vi "DOConfigureCustomaPattern.vi"(0 "object in":refnum<class "AD2_DO_SDK.lvclass">, 2 "?":T1={"DO Trigger"={"secRun(0=Cont)"=0.0, "secWait"=0.0, "cRepeat(0=inf)"=0, "Repeat Trigger"=FALSE, "TrigrSrc"=enum."trigrsrcNone"}, "CustomData"=[{"Data"=[FALSE, TRUE, FALSE, FALSE, FALSE, FALSE, FALSE, FALSE, FALSE, FALSE, FALSE, FALSE, FALSE, FALSE, FALSE, FALSE, FALSE, FALSE, FALSE, FALSE, FALSE, FALSE], "Freq"=1000.0, "#Bits"=100, "Enable"=FALSE, "IdleState"=0}, {"Data"=[TRUE, TRUE, TRUE, TRUE, TRUE, FALSE, FALSE, FALSE, FALSE, FALSE, FALSE, FALSE, FALSE, FALSE, FALSE, FALSE, FALSE, FALSE, FALSE, FALSE, FALSE, FALSE], "Freq"=1000.0, "#Bits"=100, "Enable"=FALSE, "IdleState"=0}, {"Data"=[], "Freq"=0.0, "#Bits"=0, "Enable"=FALSE, "IdleState"=0}, {"Data"=[FALSE, FALSE, FALSE, FALSE, FALSE, FALSE, FALSE, FALSE, FALSE, FALSE, FALSE, FALSE, FALSE, FALSE, FALSE, FALSE, FALSE, FALSE, FALSE, FALSE, FALSE, FALSE, FALSE], "Freq"=0.0, "#Bits"=0, "Enable"=FALSE, "IdleState"=0}, {"Data"=[], "Freq"=0.0, "#Bits"=0, "Enable"=FALSE, "IdleState"=0}, {"Data"=[], "Freq"=0.0, "#Bits"=0, "Enable"=FALSE, "IdleState"=0}, {"Data"=[], "Freq"=0.0, "#Bits"=0, "Enable"=FALSE, "IdleState"=0}, {"Data"=[], "Freq"=0.0, "#Bits"=0, "Enable"=FALSE, "IdleState"=0}, {"Data"=[], "Freq"=0.0, "#Bits"=0, "Enable"=FALSE, "IdleState"=0}, {"Data"=[], "Freq"=0.0, "#Bits"=0, "Enable"=FALSE, "IdleState"=0}, {"Data"=[], "Freq"=0.0, "#Bits"=0, "Enable"=FALSE, "IdleState"=0}, {"Data"=[], "Freq"=0.0, "#Bits"=0, "Enable"=FALSE, "IdleState"=0}, {"Data"=[], "Freq"=0.0, "#Bits"=0, "Enable"=FALSE, "IdleState"=0}, {"Data"=[], "Freq"=0.0, "#Bits"=0, "Enable"=FALSE, "IdleState"=0}, {"Data"=[], "Freq"=0.0, "#Bits"=0, "Enable"=FALSE, "IdleState"=0}, {"Data"=[FALSE, FALSE, FALSE, FALSE, FALSE, FALSE, FALSE, FALSE, FALSE, FALSE, FALSE, FALSE, FALSE, FALSE, FALSE, FALSE, FALSE, FALSE, FALSE, FALSE, FALSE, FALSE, FALSE], "Freq"=0.0, "#Bits"=0, "Enable"=FALSE, "IdleState"=0}, {"Data"=[FALSE, FALSE, FALSE, FALSE, FALSE, FALSE, FALSE, FALSE, FALSE, FALSE, FALSE, FALSE, FALSE, FALSE, FALSE, FALSE, FALSE, FALSE, FALSE, FALSE, FALSE, FALSE, FALSE], "Freq"=0.0, "#Bits"=0, "Enable"=FALSE, "IdleState"=0}]}, 5 "error in (no error)":errorcluster) -> (14 "object out":refnum<class "AD2_DO_SDK.lvclass">, 19 "error out":errorcluster)   [LabVIEW 2023, in "AD2_DO_SDK.lvclass"]
uses:
  AD2_DO_SDK.lvclass
  DOConfigureCustomData.ctl
  DOTrigger.ctl
  AD2_WFG_SDK_class/AD2TriggerSources.ctl
  DOCustomData.ctl
  AD2_DO_SDK.lvclass/AD2_DO_SDK.ctl
  Olasdwf/Olasdwf.lvlib
  AD2_SDK_class/AD2_SDK.lvclass
panel:
  out "In Range?":bool
  out "pcountOfBitsMax out":u32
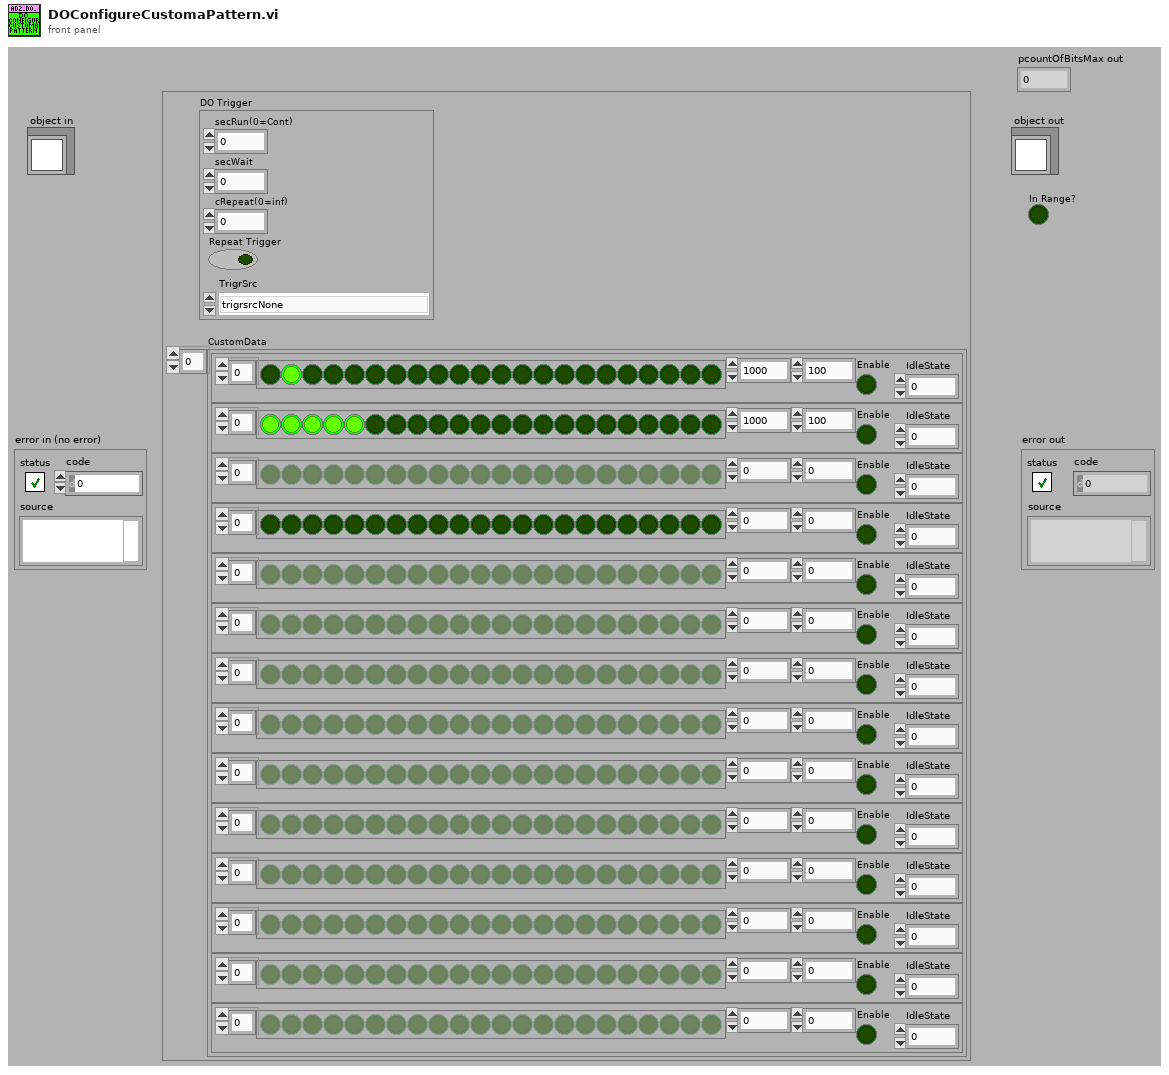
[diagram p1: front panel]
types:
  T1 = typedef "DOConfigureCustomData.ctl" = cluster{"DO Trigger":T2, "CustomData":T4}
  T2 = typedef "AD2_DO_SDK.lvclass/DOTrigger.ctl" = cluster{"secRun(0=Cont)":dbl, "secWait":dbl, "cRepeat(0=inf)":i32, "Repeat Trigger":bool, "TrigrSrc":T3}
  T3 = typedef "AD2_SDK.lvclass/AD2TriggerSources.ctl" = enum8{"trigrsrcNone", "trigsrcPC", "trigsrcDetectorAnalogIn", "trigsrcDetectorDigitalIn", "trigsrcAnalogIn", "trigsrcDigitalIn", "trigsrcDigitalOut", "trigsrcAnalogOut1", "trigsrcAnalogOut2", "trigsrcAnalogOut3", "trigsrcAnalogOut4", "trigsrcExternal1", "trigsrcExternal2", "trigsrcExternal3", "trigsrcExternal4", ""}
  T4 = typedef "AD2_DO_SDK.lvclass/DOCustomData.ctl" = cluster{"Data":bool[], "Freq":dbl, "#Bits":u32, "Enable":bool, "IdleState":u16}[]
  T5 = cluster{"NoHighBits":u32, "NoLowBits":u32, "NoInitialBits":u32, "Start High":bool}
  T6 = typedef "AD2_DO_SDK.lvclass/DOSingleCh.ctl" = cluster{"Ch Index":i32, "Enable":bool, "Clock DIvider":u32, "Type":i32, "DigitalOutOutput":u16, "IdleState":u16, "CounterData":cluster{"NoHighBits":u32, "NoLowBits":u32, "NoInitialBits":u32, "Start High":bool}, "Custom Data":cluster{"countOfBits":u32, "rgBits":u8[]}}
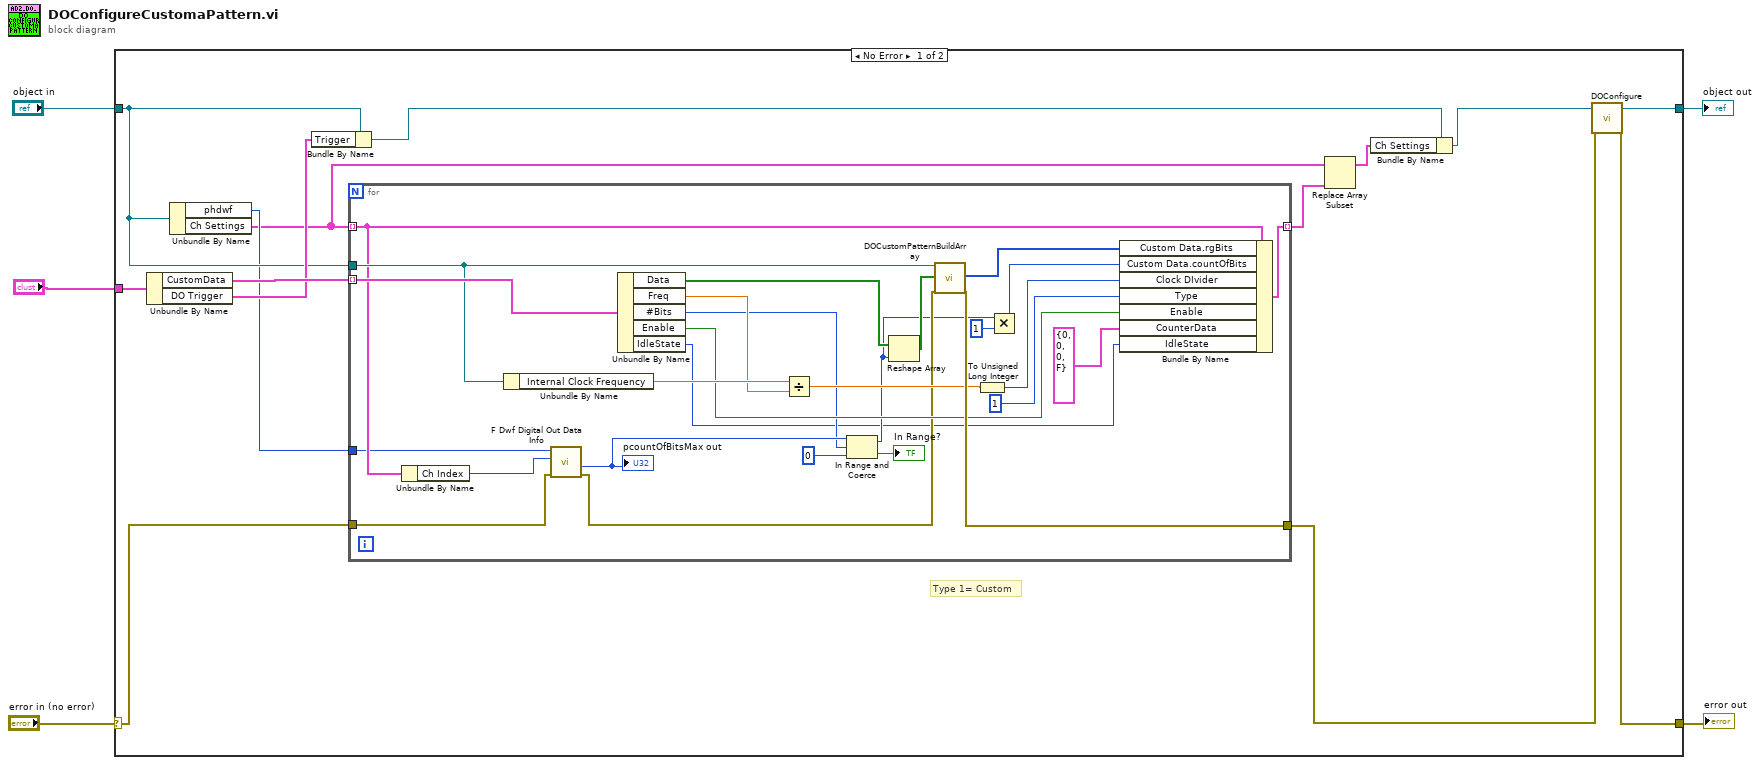
[diagram p0: block diagram]
diagram:
  n1 = case shown="No Error" "error in (no error)" {
    selector: "error in (no error)" -> [w13 w48]
    tunnel: [w19 w48] -> w4
    tunnel: [w18 w47] -> w2
    tunnel: "object in" -> [w10 w47]
    tunnel: "?" -> [w15 _]
    frame No Error {
      # "Type 1= Custom"
      n2 = Unbundle By Name(w15) -> ("CustomData"=w14:T4, "DO Trigger"=w12:T2)
      n3 = Unbundle By Name(w10) -> ("phdwf"=w9:i32, "Ch Settings"=w8:T6[])
      n4 = Bundle By Name(cluster=w10, "Trigger"=w12) -> (w11:refnum<class "AD2_DO_SDK.lvclass">)
      n5 = for {
        tunnel: w8 -> [w30] mode=indexing
        tunnel: [w46] -> w7 mode=indexing
        tunnel: w14 -> [w39] mode=indexing
        tunnel: w13 -> [w26]
        tunnel: [w44] -> w16
        tunnel: w10 -> [w38]
        tunnel: w9 -> [w29]
        n6 = Unbundle By Name(w30) -> ("Ch Index"=w28:i32)
        n7 = Unbundle By Name(w38) -> ("Internal Clock Frequency"=w37:dbl)
        n8 = call "F Dwf Digital Out Data Info.vi"("error in (no error)"=w26, "idxChannel"=w28, "hdwf"=w29) -> ("error out"=w27:errorcluster, "pcountOfBitsMax out"=w25:u32)  [unwired: 6 in, 1 out]
        "pcountOfBitsMax out" <- w25
        n9 = Unbundle By Name(w39) -> ("Data"=w43:bool[], "Freq"=w36:dbl, "#Bits"=w22:u32, "Enable"=w32:bool, "IdleState"=w20:u16)
        n10 = Divide(x=w37, y=w36) -> (x/y=w35:dbl)
        n11 = In Range and Coerce(upper limit=w25, x=w22, lower limit=u32 0) -> (coerced(x)=w21:u32, In Range?=→"In Range?":bool)
        n12 = Reshape Array(w43, w21) -> (w42:bool[])
        n13 = call-dynamic "DOCustomPatternBuildArray.vi"("object in"=w38, "Data"=w42, "error in (no error)"=w27) -> ("Array"=w45:u8[], "error out"=w44:errorcluster)  [unwired: 14 in, 1 out]
        n14 = To Unsigned Long Integer(number=w35) -> (unsigned 32bit integer=w34:u32)
        n15 = Multiply(x=w21, y=u32 1) -> (x*y=w40:u32)
        n16 = Bundle By Name(cluster=w30, "Custom Data.rgBits"=w45, "Custom Data.countOfBits"=w40, "Clock DIvider"=w34, "Type"=1, "Enable"=w32, "CounterData"=T5 {"NoHighBits"=0, "NoLowBits"=0, "NoInitialBits"=0, "Start High"=FALSE}, "IdleState"=w20) -> (w46:T6)
      }
      n17 = Replace Array Subset(array=w8, new element=w7) -> (w6:T6[])  [unwired: 1 in]
      n18 = Bundle By Name(cluster=w11, "Ch Settings"=w6) -> (w17:refnum<class "AD2_DO_SDK.lvclass">)
      n19 = call-dynamic "DOConfigure.vi"("object in"=w17, "error in (no error)"=w16) -> ("object out"=w18:refnum<class "AD2_DO_SDK.lvclass">, "error out"=w19:errorcluster)  [unwired: 16 in]
    }
    frame Error {
    }
  }
  "error out" <- w4
  "object out" <- w2
